vi "Read module.vi"(8 "error in (no error)":errorcluster, 11 "IDLFile in":refnum<class "IDLFile.lvclass">) -> (0 "error out":errorcluster, 2 "Module.lvclass":refnum<class "Module.lvclass">, 3 "IDLFile out":refnum<class "IDLFile.lvclass">)   [LabVIEW 2018, in "IDLFile.lvclass"]
doc: "Read the module."
uses:
  IDLFile.lvclass
  Module/Module.lvclass
  IDLFile.lvclass/IDLFile.ctl
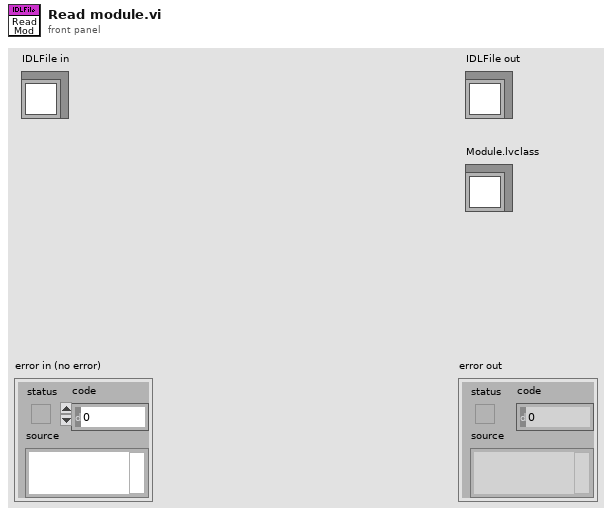
[diagram p1: front panel]
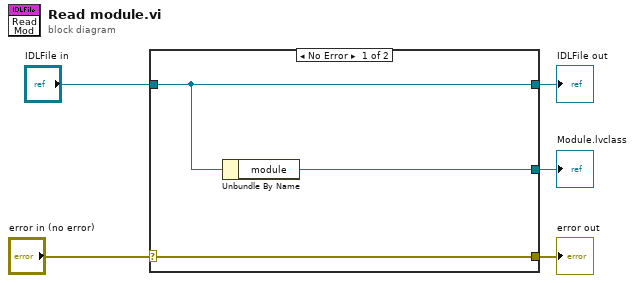
[diagram p0: block diagram]
diagram:
  n1 = case shown="No Error" "error in (no error)" {
    selector: "error in (no error)" -> [w8 w9]
    tunnel: [w8 w9] -> w4
    tunnel: [w7 w10] -> w2
    tunnel: "IDLFile in" -> [w7 w10]
    tunnel: [w6 _] -> w1
    frame No Error {
      n2 = Unbundle By Name(w7) -> ("module"=w6:refnum<class "Module.lvclass">)
    }
    frame Error {
    }
  }
  "error out" <- w4
  "IDLFile out" <- w2
  "Module.lvclass" <- w1
